vi "Scalar JSON text to Variant.vi"(6 "Type":T1, 8 "error in (no error)":errorcluster, 9 "Variant (Data Type)":variant, 10 "Offset":i32, 11 "JSON":string) -> (0 "error out":errorcluster, 1 "Variant out":variant)   [LabVIEW 2017, in "JSONtext.lvlib"]
uses:
  JSONtext.lvlib
  <vilib>/Utility/Data Type/Type Definitions/Data Type.ctl
  <vilib>/Utility/Data Type/Type Definitions/Refnum Type.ctl
  Advance past String.vi
  String Subset.vi
  support/Strip Quotes and Unescape.vi
  support/Format Error.vi
  support/Get Number Text.vi
  NaN or null to Integer ERROR.vi
  Advance past Number.vi
  Parsing Error.vi
  support/Unescape JSON string.vi
  support/Scan Timestamp.vi
  <vilib>/Utility/Data Type/NI_Data Type.lvlib
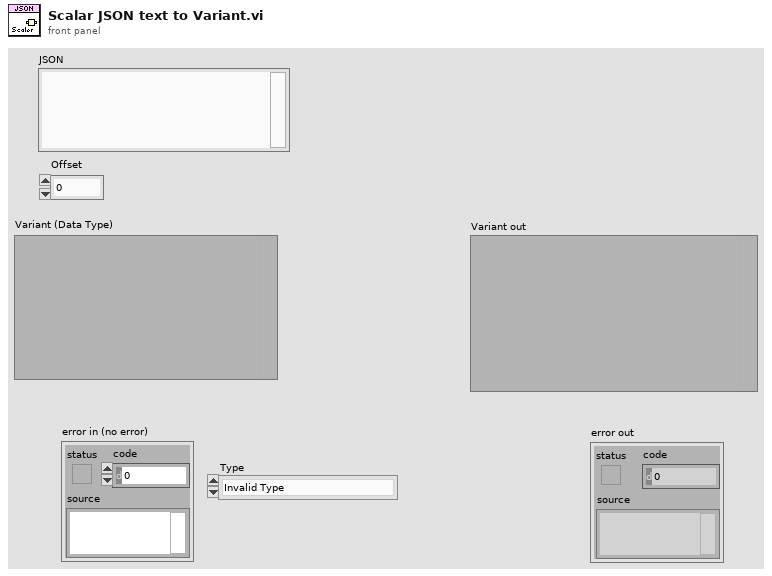
[diagram p1: front panel]
types:
  T1 = typedef "NI_Data Type.lvlib/Data Type.ctl" = enum8{"Invalid Type", "Void", "I8", "I16", "I32", "I64", "U8", "U16", "U32", "U64", "Single Float", "Double Float", "Extended Float", "Single Complex", "Double Complex", "Extended Complex", "Enum U8", "Enum U16", "Enum U32", "Enum U64", "Single Float With Unit", "Double Float With Unit", "Extended Float With Unit", "Single Complex with Unit", "Double Complex with Unit", "Extended Complex with Unit", "Boolean", "String", "Path", "Picture", "Tag", "Array", "Cluster", "Variant", "LV Variant", "Waveform", "Timestamp", "Digital Waveform", "Digital Data", "ExpressData", "Refnum", "External Data", "VI", "Poly VI", "LabVIEW Class Instance", "Fixed Point"}
  T2 = typedef "JSONtext.lvlib/Parsing State.ctl" = enum16{"Parser Error", "Object", "Array", "String", "Number/Other", "Leading Whitespace", "Object end", "Array end", "Value end"}
  T3 = typedef "NI_Data Type.lvlib/Refnum Type.ctl" = enum16{"NotARefnum", "UnknownRefnum", "Generic", "Datalog", "ByteStream", "Device", "Occurence", "TCPNetConnection", "Auto", "Menu", "Imaq", "Hardware", "DataSocket", "Visa", "IVI", "UDPNetConnection", "Notifier", "Queue", "Irda", "EventReg", "DotNet", "UserEvent", "Callback", "UNUSED_EMPTY_POSITION", "BlueToothNetConnection", "LVObjApp", "LVObjVI", "LVObjUnknown", "GenericClass", "UserDefinedRefnumTag", "DataValue", "RT FIFO", "TDMS File"}
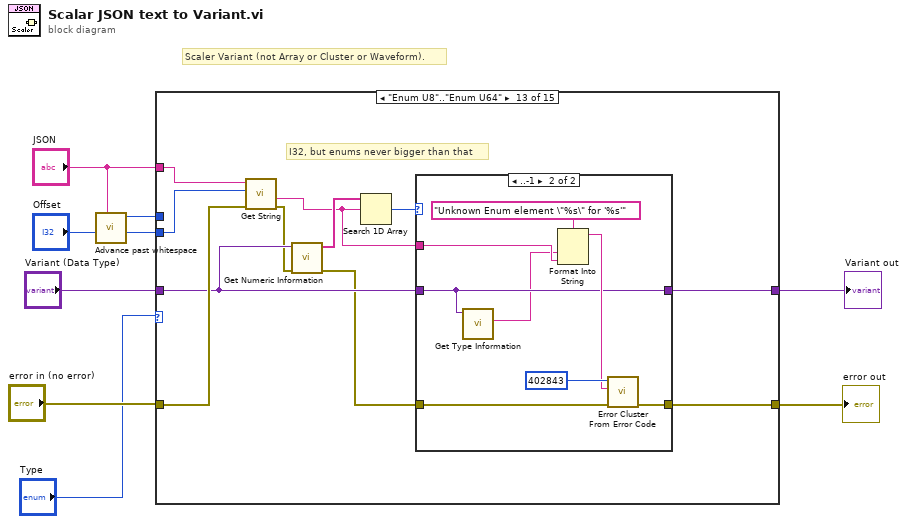
[diagram p0: block diagram]
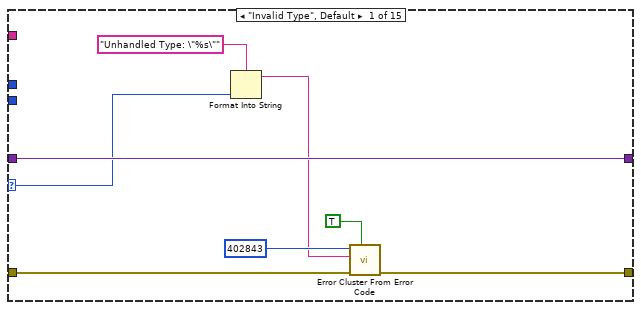
[diagram p2: hidden frame]
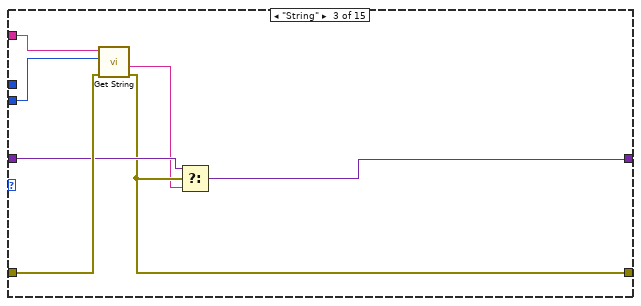
[diagram p4: hidden frame]
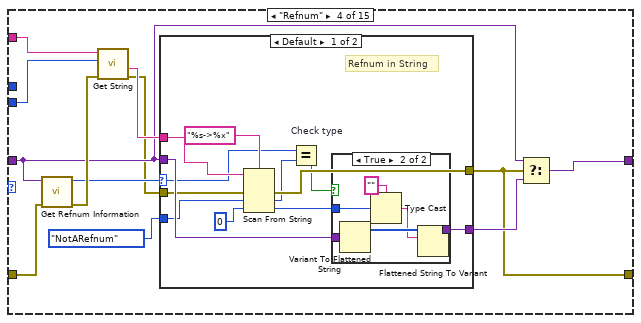
[diagram p5: hidden frame]
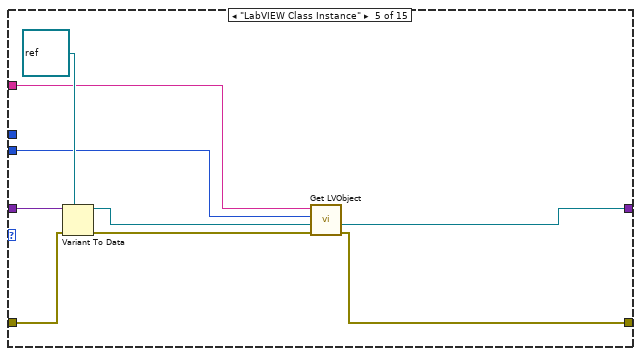
[diagram p8: hidden frame]
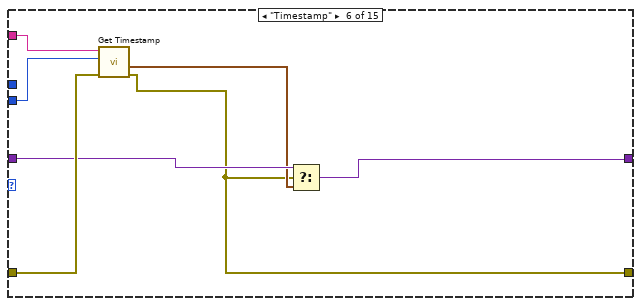
[diagram p9: hidden frame]
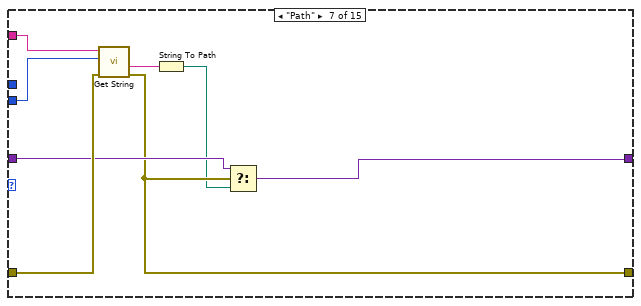
[diagram p10: hidden frame]
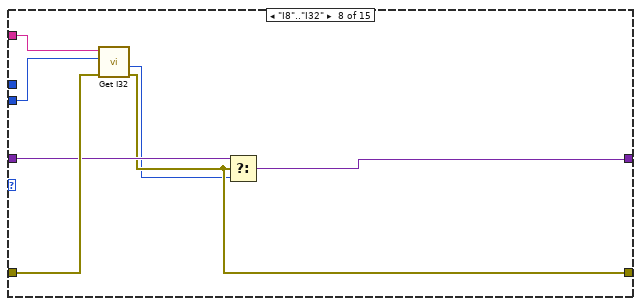
[diagram p11: hidden frame]
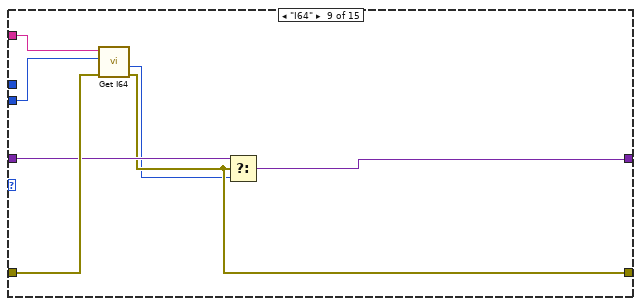
[diagram p12: hidden frame]
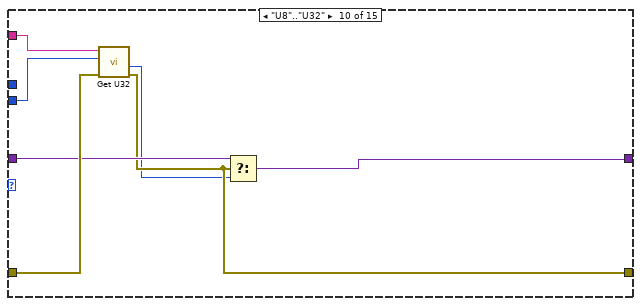
[diagram p13: hidden frame]
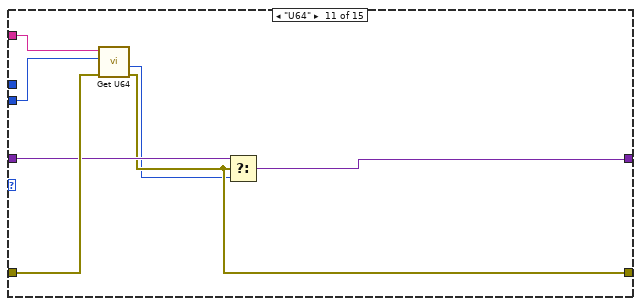
[diagram p14: hidden frame]
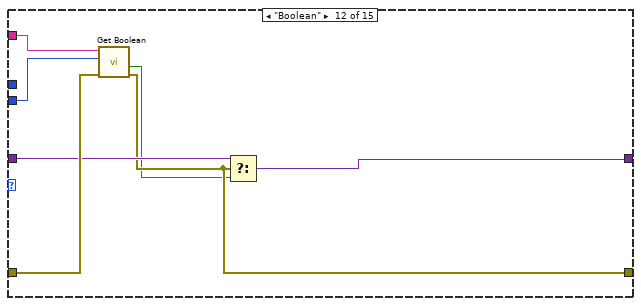
[diagram p15: hidden frame]
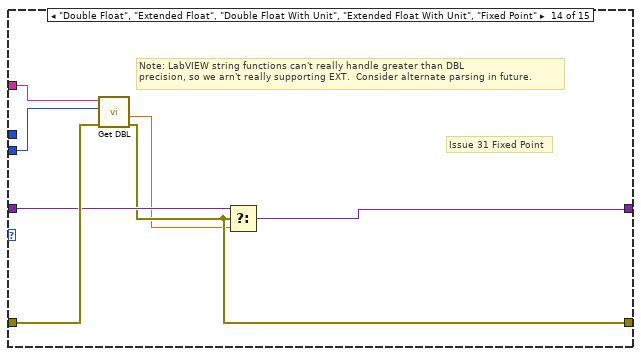
[diagram p17: hidden frame]
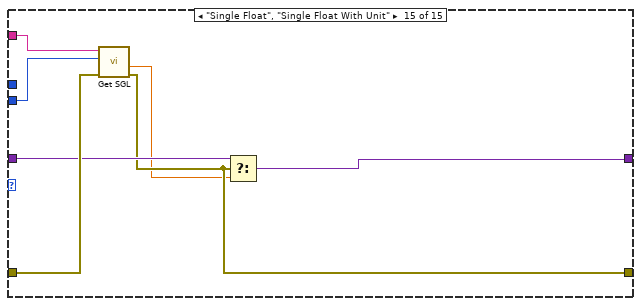
[diagram p18: hidden frame]
diagram:
  # "Scaler Variant (not Array or Cluster or Waveform)."
  n1 = call "Advance past whitespace.vi"("JSON"="JSON", "Offset"="Offset") -> ("Offset of first non-whitespace"=w5:i32, "Parser State"=w3:T2)  [unwired: 8 in]
  n2 = case shown="\"Enum U8\"..\"Enum U64\"" "Type" {
    selector: "Type" -> [w12 _ _ _ _ _ _ _ _ _ _ _ _ _ _]
    tunnel: "Variant (Data Type)" -> [w16 w18 w23 w30 w67 w72 w80 w88 w95 w102 w109 w116 w123 w144 w151]
    tunnel: "JSON" -> [_ _ w25 w37 w61 w74 w82 w85 w92 w99 w106 w113 w127 w141 w148]
    tunnel: [w15 w19 w21 w28 w66 w69 w78 w86 w93 w100 w107 w114 w122 w142 w149] -> w8
    tunnel: "error in (no error)" -> [w17 w19 w24 w35 w65 w73 w81 w89 w96 w103 w110 w117 w128 w145 w152]
    tunnel: w5 -> [_ _ w26 w38 w62 w75 w83 w90 w97 w104 w111 w118 w129 w146 w153]
    tunnel: [w16 w18 w22 w36 w60 w71 w79 w87 w94 w101 w108 w115 w124 w143 w150] -> w7
    tunnel: w3 -> [_ _ _ _ _ _ _ _ _ _ _ _ _ _ _]
    frame "Invalid Type", Default {
      n3 = Format Into String(format string="Unhandled Type: \"%s\"", w12) -> (resulting string=w10:string)  [unwired: 2 in, 1 out]
      n4 = call <vilib>:"Error Cluster From Error Code.vi"("show call chain? (False)"=TRUE, "error in (no error)"=w17, "error message (\"\")"=w10, "error code (0)"=402843) -> ("error out"=w15:errorcluster)  [unwired: 5 in]
    }
    frame "Void" {
      # "Empty Variant: #ToDo Variant Attributes?"
    }
    frame "String" {
      n5 = call "Get String.vi"("error in (no error)"=w24, "Offset"=w26, "JSON"=w25) -> ("error out"=w21:errorcluster, "String"=w20:string)  [unwired: 6 in, 1 out]
      n6 = Select(t=w23, s=w21, f=w20) -> (s? t:f=w22:variant)
    }
    frame "Refnum" {
      n7 = call <vilib>:"Get Refnum Information.vi"("error in (no error)"=w35, "Variant"=w30) -> ("error out"=w34:errorcluster, "Reference Type"=w33:T3)  [unwired: 6 in, 2 out]
      n8 = call "Get String.vi"("error in (no error)"=w34, "Offset"=w38, "JSON"=w37) -> ("error out"=w29:errorcluster, "String"=w31:string)  [unwired: 6 in, 1 out]
      n9 = case shown="Default" w33 {
        selector: w33 -> [w39 _]
        tunnel: [w49 w59] -> w32
        tunnel: w31 -> [w43 w59]
        tunnel: w30 -> [w50 _]
        tunnel: w29 -> [w45 w58]
        tunnel: [w44 w58] -> w28
        tunnel: Refnum_Type."NotARefnum" ("Reference Type") -> [w42 _]
        frame Default {
          # "Refnum in String"
          n10 = Scan From String(format string="%s->%x", input string=w43, error in=w45, default 1=w42, default 2=u32 0) -> (error out=w44:errorcluster, output 1=w41:T3, output 2=w46:u32)  [unwired: 1 in, 2 out]
          n11 = Equal? "Check type"(x=w39, y=w41) -> (x = y?=w40:bool)
          n12 = case shown="True" w40 {
            tunnel: w50 -> [w51 w55]
            tunnel: [w51 w54] -> w49
            tunnel: w46 -> [_ w52]
            frame False {
            }
            frame True {
              n13 = Variant To Flattened String(Variant=w55) -> (1:w57:i16[])  [unwired: 1 out]
              n14 = Type Cast(type="", x=w52) -> (*(type *) &x=w56:string)
              n15 = Flattened String To Variant(6:w56, 7:w57) -> (3:w54:variant)  [unwired: 1 in, 1 out]
            }
          }
        }
        frame "Visa", "IVI", "UserDefinedRefnumTag" {
        }
      }
      n16 = Select(t=w30, s=w28, f=w32) -> (s? t:f=w36:variant)
    }
    frame "LabVIEW Class Instance" {
      n17 = Variant To Data(error in=w65, type=refnum<class> refnum ("LabVIEW Object"), Variant=w67) -> (data=w63:refnum<class>, error out=w64:errorcluster)
      n18 = call "Get LVObject.vi"("error in (no error)"=w64, "Object Type"=w63, "Offset"=w62, "JSON String containing Flattened Object"=w61) -> ("error out"=w66:errorcluster, "Object out"=w60:refnum<class>)  [unwired: 5 in, 1 out]
    }
    frame "Timestamp" {
      n19 = call "Get Timestamp.vi"("error in (no error)"=w73, "Offset"=w75, "JSON"=w74) -> ("error out"=w69:errorcluster, "Timestamp"=w70:timestamp)  [unwired: 6 in, 1 out]
      n20 = Select(t=w72, s=w69, f=w70) -> (s? t:f=w71:variant)
    }
    frame "Path" {
      n21 = call "Get String.vi"("error in (no error)"=w81, "Offset"=w83, "JSON"=w82) -> ("error out"=w78:errorcluster, "String"=w76:string)  [unwired: 6 in, 1 out]
      n22 = String To Path(string=w76) -> (path=w77:path)
      n23 = Select(t=w80, s=w78, f=w77) -> (s? t:f=w79:variant)
    }
    frame "I8".."I32" {
      n24 = call "Get I32.vi"("error in (no error)"=w89, "Offset"=w90, "JSON"=w85) -> ("error out"=w86:errorcluster, "Number"=w84:i32)  [unwired: 6 in, 1 out]
      n25 = Select(t=w88, s=w86, f=w84) -> (s? t:f=w87:variant)
    }
    frame "I64" {
      n26 = call "Get I64.vi"("error in (no error)"=w96, "Offset"=w97, "JSON"=w92) -> ("error out"=w93:errorcluster, "Number"=w91:i64)  [unwired: 6 in, 1 out]
      n27 = Select(t=w95, s=w93, f=w91) -> (s? t:f=w94:variant)
    }
    frame "U8".."U32" {
      n28 = call "Get U32.vi"("error in (no error)"=w103, "Offset"=w104, "JSON"=w99) -> ("error out"=w100:errorcluster, "Number"=w98:u32)  [unwired: 6 in, 1 out]
      n29 = Select(t=w102, s=w100, f=w98) -> (s? t:f=w101:variant)
    }
    frame "U64" {
      n30 = call "Get U64.vi"("error in (no error)"=w110, "Offset"=w111, "JSON"=w106) -> ("error out"=w107:errorcluster, "Number"=w105:u64)  [unwired: 6 in, 1 out]
      n31 = Select(t=w109, s=w107, f=w105) -> (s? t:f=w108:variant)
    }
    frame "Boolean" {
      n32 = call "Get Boolean.vi"("error in (no error)"=w117, "Offset"=w118, "JSON"=w113) -> ("error out"=w114:errorcluster, "Boolean"=w112:bool)  [unwired: 6 in, 1 out]
      n33 = Select(t=w116, s=w114, f=w112) -> (s? t:f=w115:variant)
    }
    frame "Enum U8".."Enum U64" {
      # "I32, but enums never bigger than that"
      n34 = call "Get String.vi"("error in (no error)"=w128, "Offset"=w129, "JSON"=w127) -> ("error out"=w120:errorcluster, "String"=w121:string)  [unwired: 6 in, 1 out]
      n35 = call <vilib>:"Get Numeric Information.vi"("error in (no error)"=w120, "Variant"=w123) -> ("error out"=w119:errorcluster, "Enum Names"=w125:string[])  [unwired: 6 in, 2 out]
      n36 = Search 1D Array(1D array=w125, element=w121) -> (index of element=w126:i32)  [unwired: 1 in]
      n37 = case shown="..-1" w126 {
        selector: w126 -> [w130 _]
        tunnel: [w130 w133] -> w124
        tunnel: w123 -> [_ w133]
        tunnel: w119 -> [w131 w137]
        tunnel: [w131 w139] -> w122
        tunnel: w121 -> [_ w136]
        frame 0.. {
        }
        frame ..-1 {
          n38 = call <vilib>:"Get Type Information.vi"("Variant"=w133) -> ("Name"=w132:string)  [unwired: 6 in, 4 out]
          n39 = Format Into String(format string="Unknown Enum element \"%s\" for '%s'", w132, w136) -> (resulting string=w134:string)  [unwired: 2 in, 1 out]
          n40 = call <vilib>:"Error Cluster From Error Code.vi"("error in (no error)"=w137, "error message (\"\")"=w134, "error code (0)"=402843) -> ("error out"=w139:errorcluster)  [unwired: 6 in]
        }
      }
    }
    frame "Double Float", "Extended Float", "Double Float With Unit", "Extended Float With Unit", "Fixed Point" {
      # "Issue 31 Fixed Point"
      # "Note: LabVIEW string functions can't really handle greater than DBL\nprecision, so we arn't really supporting EXT.  Consider alternate parsing in future."
      n41 = call "Get DBL.vi"("error in (no error)"=w145, "Offset"=w146, "JSON"=w141) -> ("error out"=w142:errorcluster, "Number"=w140:dbl)  [unwired: 6 in, 1 out]
      n42 = Select(t=w144, s=w142, f=w140) -> (s? t:f=w143:variant)
    }
    frame "Single Float", "Single Float With Unit" {
      n43 = call "Get SGL.vi"("error in (no error)"=w152, "Offset"=w153, "JSON"=w148) -> ("error out"=w149:errorcluster, "Number"=w147:sgl)  [unwired: 6 in, 1 out]
      n44 = Select(t=w151, s=w149, f=w147) -> (s? t:f=w150:variant)
    }
  }
  "Variant out" <- w7
  "error out" <- w8
